vi "searchForaString.vi"() -> ()   [LabVIEW 2021]
uses:
  <vilib>/Utility/file.llb/Read Delimited Spreadsheet (string).vi
panel:
  in  "String":string
  out "sum":i16
  out "all rows":string[][](array[string])
  in  "file path (dialog if empty)":path
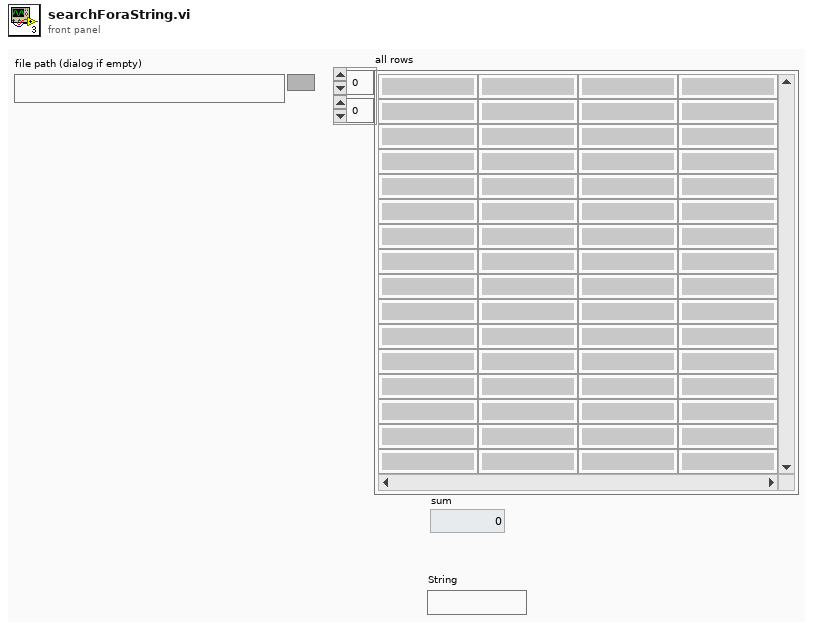
[diagram p1: front panel]
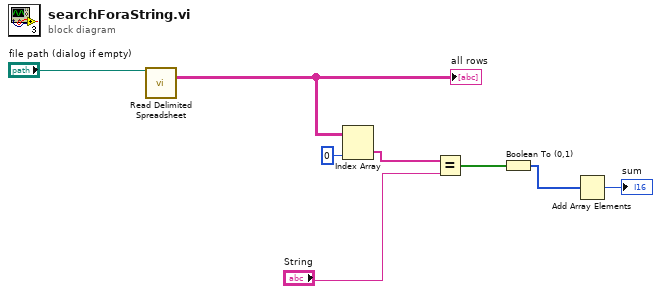
[diagram p0: block diagram]
diagram:
  n1 = call-poly <vilib>:"Read Delimited Spreadsheet.vi"("file path (dialog if empty)"="file path (dialog if empty)") -> ("all rows"=w7:string[][])  [unwired: 9 in, 5 out]
  "all rows" <- w7
  n2 = Index Array(array=w7, index (col)=0 ("disabled index (col)")) -> (element=w5:string[])  [unwired: 1 in]
  n3 = Equal?(x=w5, y="String") -> (x = y?=w4:bool[])
  n4 = Boolean To (0,1)(Boolean=w4) -> (0, 1=w3:i16[])
  n5 = Add Array Elements(numeric array=w3) -> (sum=→"sum":i16)
